vi "configure operation.vi"(7 "tag bus configurable plugin module configuration":refnum<class "io configuration.lvclass">, 8 "error in":errorcluster, 10 "line item in":T3, 11 "engine configuration":refnum<class "engine configuration.lvclass">) -> (0 "error out":errorcluster, 1 "success":bool, 2 "line item out":T3, 5 "changed":bool)   [LabVIEW 2017, in "io editor node.lvclass"]
uses:
  io editor node.lvclass
  table line.ctl
  <vilib>/NI/Tag Bus Module Framework/channel/TBM channel.lvclass
  C:/Program Files (x86)/National Instruments/LabVIEW 2017/vi.lib/NI/Tag Bus/tag/tag descriptor.lvclass
  <vilib>/NI/Module Execution Interface/Engine Configuration/engine configuration.lvclass
  permissions.ctl
  configuration/io configuration.lvclass
  C:/Program Files (x86)/National Instruments/LabVIEW 2017/vi.lib/NI/Configuration Framework/serializable configuration/NISE_CEF_serializable configuration.lvclass
  source/fifo channel/fifo channel settings.ctl
  source/fifo channel/fifo channel.lvclass
  C:/Program Files (x86)/National Instruments/LabVIEW 2017/vi.lib/NI/Tag Bus Module Framework/channel/TBM channel.lvclass
  source/fifo channel/fifo channel.lvclass/fifo channel.ctl
  <vilib>/NI/Tag Bus Module Framework/channel/TBM channel.lvclass/TBM channel.ctl
  <vilib>/NI/Tag Bus/tag/tag descriptor.lvclass/tag descriptor.ctl
  <vilib>/NI/Configuration Framework/serializable configuration/NISE_CEF_serializable configuration.lvclass/NISE_CEF_serializable configuration.ctl
  source/fifo channel/Read fifo config.vi
  <vilib>/NI/Tag Bus Module Framework/channel/Read channel classification.vi
  <vilib>/NI/Tag Bus/tag/read data type.vi
  <vilib>/NI/Configuration Framework/serializable configuration/Read UID.vi
  <vilib>/NI/Tag Bus/tag/write tag name.vi
  source/fifo channel/Write fifo config.vi
  <vilib>/NI/Tag Bus/tag/write data type.vi
  <vilib>/NI/Tag Bus Module Framework/channel/Write channel classification.vi
  <vilib>/Utility/LVClass/Get LV Class Name.vi
  <vilib>/NI/Configuration Framework/error generator/NISE_error generator.vi
  <vilib>/NI/Tag Bus/tag/tag descriptor.lvclass
panel:
  in  "fifo config":T1
  out "errors":string
  in  "Access Type":T2
  in  "Tag":i32(listbox)
  in  "Data Type":i32(listbox)
  in  "Terminal Label":string
  in  "cancel":bool
  in  "ok":bool
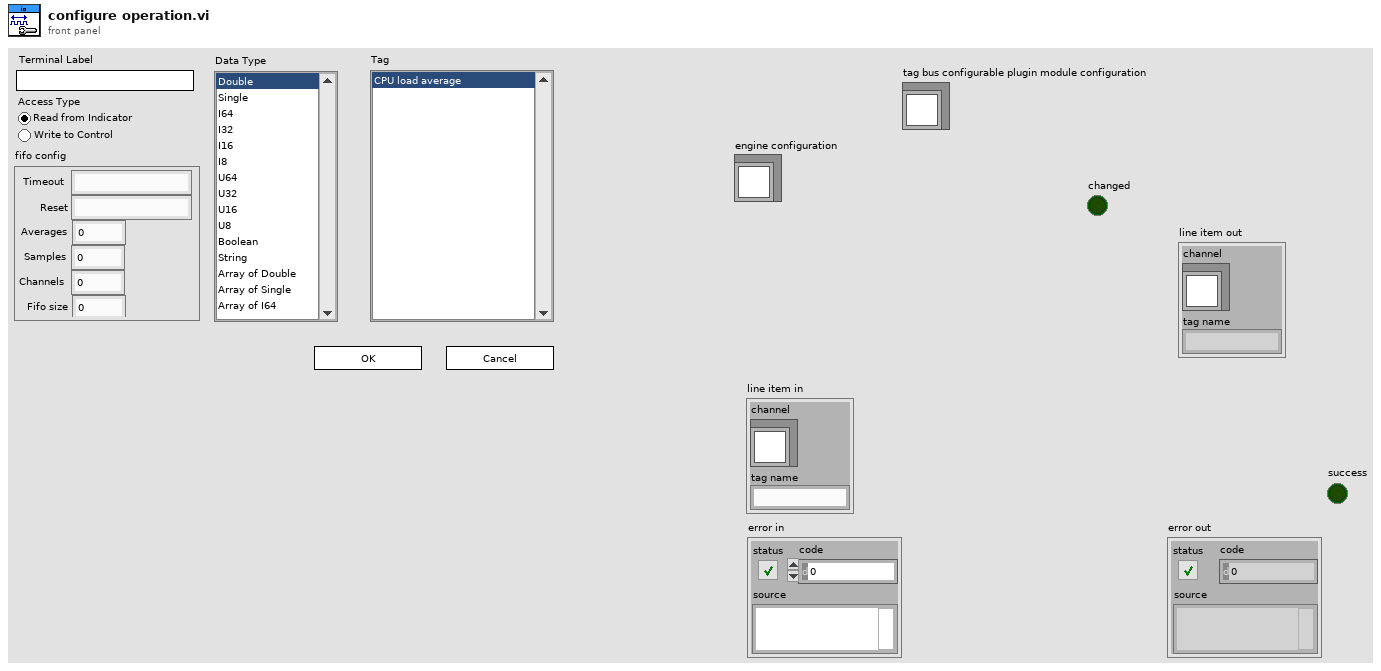
[diagram p1: front panel]
types:
  T1 = typedef "fifo channel.lvclass/fifo channel settings.ctl" = cluster{"Timeout":string, "Reset":string, "Averages":i32, "Samples":u32, "Channels":i32, "Fifo size":u32}
  T2 = typedef "io editor node.lvclass/permissions.ctl" = enum32{"Read from Indicator", "Write to Control"}
  T3 = typedef "io editor node.lvclass/table line.ctl" = cluster{"channel":refnum<class "TBM channel.lvclass">, "tag name":string}
  T4 = enum32{"Invalid", "Standard", "Closed", "Hidden", "Minimized", "Maximized"}
  T5 = enum32{"Invalid", "Default", "Floating", "Floating/Auto-Hide", "Modal"}
  T6 = enum8{"Enabled", "Disabled", "Disabled and Grayed Out"}
  T7 = enum32{"invalid app kind", "Development System", "Run Time System", "Student Edition", "Embedded LabVIEW", "Evaluation", "Custom"}
  T8 = typedef "tag bus.lvlib/tag descriptor.lvclass/Data Type.ctl" = enum16{"Double", "Single", "I64", "I32", "I16", "I8", "U64", "U32", "U16", "U8", "Boolean", "String", "Array of Double", "Array of Single", "Array of I64", "Array of I32", "Array of I16", "Array of I8", "Array of U64", "Array of U32", "Array of U16", "Array of U8", "Array of Boolean", "Array of String"}
  T9 = typedef "TBM channel.lvclass/channel classification.ctl" = enum16{"input data", "output data", "processing parameter", "processing result"}
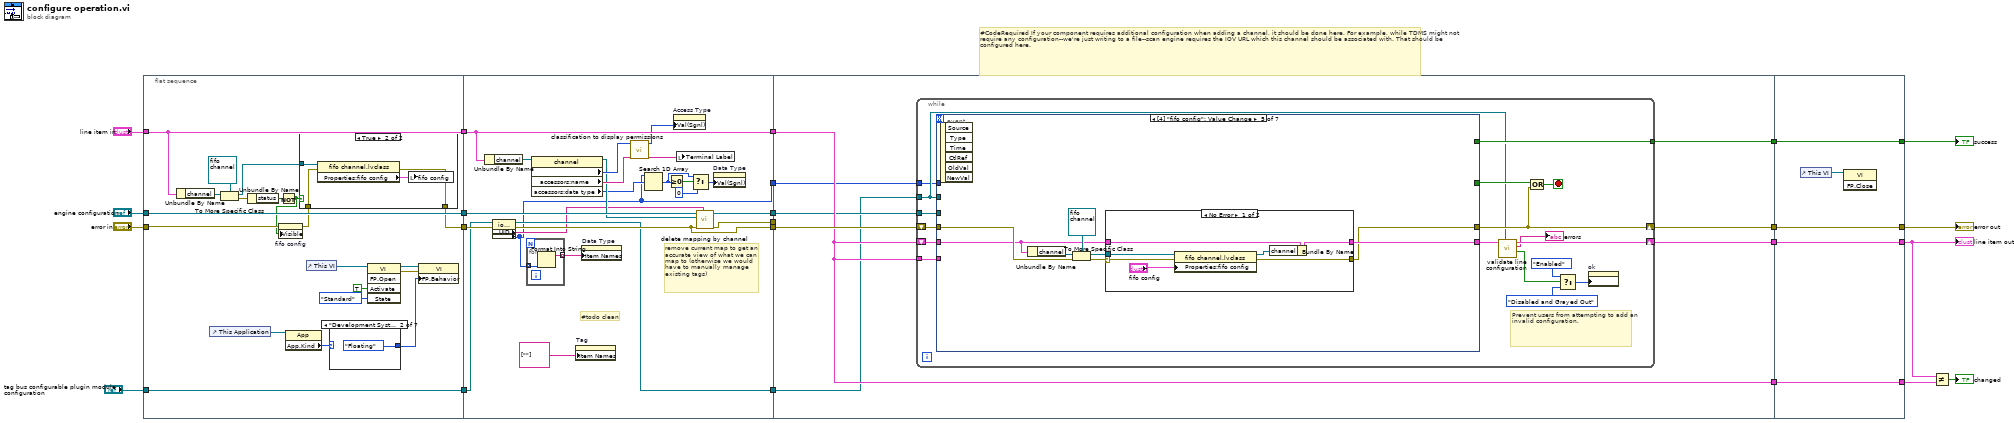
[diagram p0: block diagram]
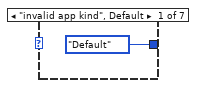
[diagram p3: hidden frame]
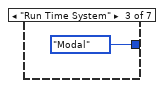
[diagram p4: hidden frame]
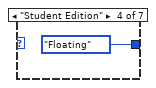
[diagram p5: hidden frame]
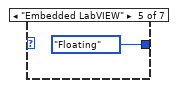
[diagram p6: hidden frame]
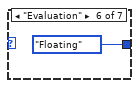
[diagram p7: hidden frame]
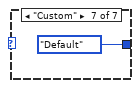
[diagram p8: hidden frame]
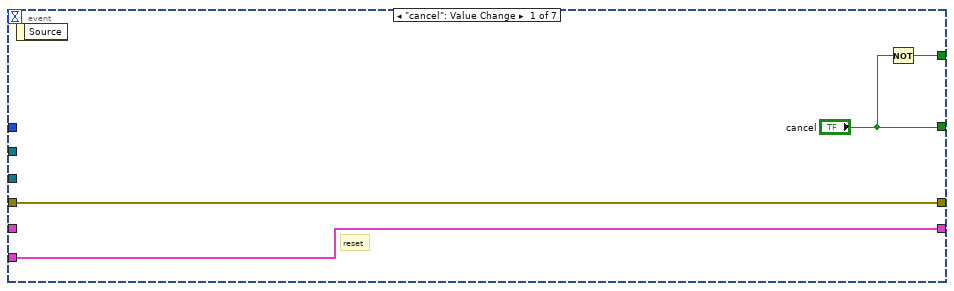
[diagram p9: hidden frame]
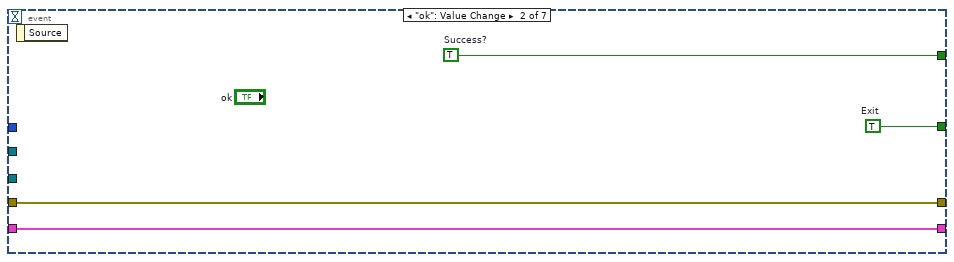
[diagram p10: hidden frame]
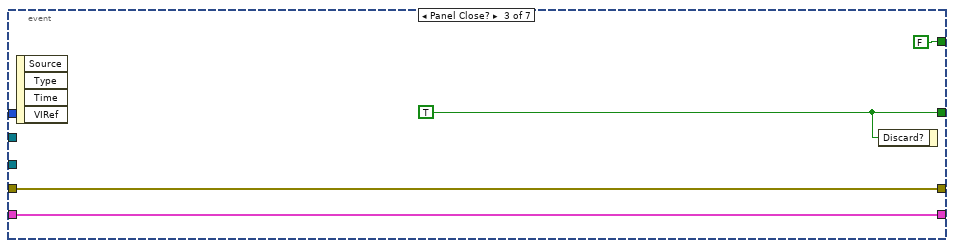
[diagram p11: hidden frame]
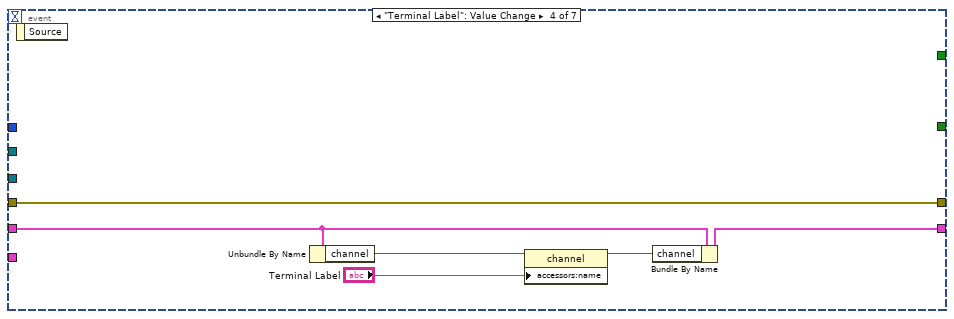
[diagram p12: hidden frame]
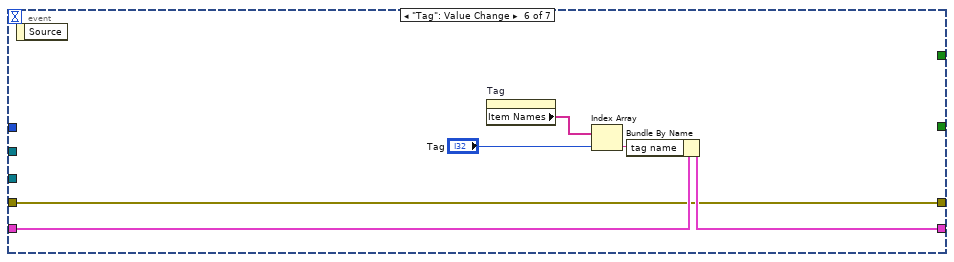
[diagram p14: hidden frame]
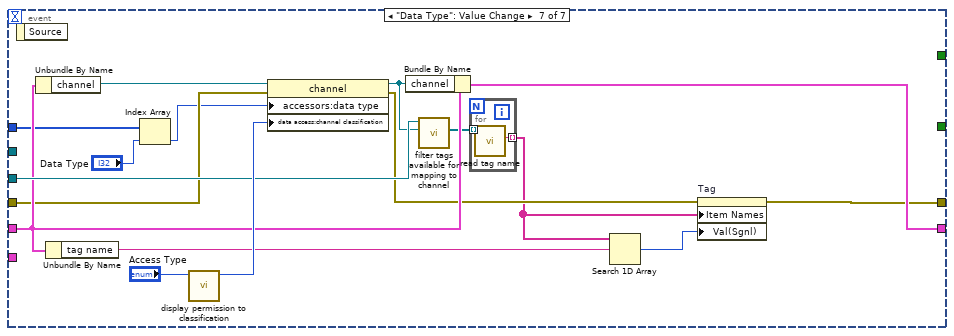
[diagram p15: hidden frame]
diagram:
  # "#CodeRequired If your component requires additional configuration when adding a channel, it should be done here. For example, while TDMS might not require any configuration--we're just writing to a file--scan engine requires the IOV URL which this channel should be associated with. That should be configured here."
  n1 = flat-sequence {
    tunnel: "line item in" -> [w33]
    tunnel: "error in" -> [w26]
    tunnel: [w28] -> w12
    tunnel: [w33] -> w11
    tunnel: [w35] -> w8
    tunnel: "engine configuration" -> [w35]
    tunnel: [w34] -> w5
    tunnel: "tag bus configurable plugin module configuration" -> [w34]
    tunnel: w12 -> [w69]
    tunnel: w11 -> [w74]
    tunnel: [w74] -> w10
    tunnel: [w72] -> w9
    tunnel: w8 -> [w73]
    tunnel: [w66] -> w6
    tunnel: w5 -> [w67]
    tunnel: [w68] -> w4
    tunnel: [w70] -> w3
    tunnel: [w56] -> w2
    tunnel: [w86] -> w16
    tunnel: [w85] -> w15
    tunnel: [w84] -> w14
    tunnel: [w83] -> w13
    tunnel: w10 -> [w83]
    tunnel: w9 -> [w82]
    tunnel: w6 -> [w81]
    tunnel: w4 -> [w87]
    tunnel: w3 -> [_]
    tunnel: w2 -> [w80]
    tunnel: [w166] -> w17
    tunnel: [w167] -> w20
    tunnel: [w168] -> w21
    tunnel: [w169] -> w22
    tunnel: w16 -> [w169]
    tunnel: w15 -> [w168]
    tunnel: w14 -> [w167]
    tunnel: w13 -> [w166]
    frame #0 {
      n2 = Unbundle By Name(w33) -> ("channel"=w32:refnum<class "TBM channel.lvclass">)
      n3 = control-ref of="This Application"() -> (w38:refnum<vi>)
      n4 = To More Specific Class(target class=refnum<class "fifo channel.lvclass"> refnum ("fifo channel.lvclass"), reference=w32) -> (specific class reference=w27:refnum<class "fifo channel.lvclass">, error out=w30:errorcluster)  [unwired: 1 in]
      n5 = Unbundle By Name(w30) -> ("status"=w29:bool)
      n6 = Not(x=w29) -> (.not. x?=w24:bool)
      n7 = property on="fifo config" class="Clust (strict)"(error in=w26, "Visible"=w24) -> (error out=w25:errorcluster)  [unwired: 1 in, 1 out]
      n8 = property class="App"(reference=w38) -> ("App.Kind"=w37:T7)  [unwired: 1 in, 2 out]
      n9 = case shown="True" w24 {
        tunnel: w25 -> [w44 w47]
        tunnel: [w44 w45] -> w28
        tunnel: w27 -> [_ w48]
        frame False {
        }
        frame True {
          n10 = property class="fifo channel.lvclass"(reference=w48, error in=w47) -> (error out=w45:errorcluster, "Properties:fifo config"=w46:T1)  [unwired: 1 out]
          n11 = local write "fifo config"(w46) -> ()
        }
      }
      n12 = control-ref of="This VI"() -> (w39:refnum<vi>)
      n13 = case shown="\"Development System\"" w37 {
        tunnel: [T5."Default" ("Front Panel Window:Behavior") T5."Floating" ("Front Panel Window:Behavior") T5."Modal" ("Front Panel Window:Behavior") T5."Floating" ("Front Panel Window:Behavior") T5."Floating" ("Front Panel Window:Behavior") T5."Floating" ("Front Panel Window:Behavior") T5."Default" ("Front Panel Window:Behavior")] -> w36
        frame "invalid app kind", Default {
        }
        frame "Development System" {
        }
        frame "Run Time System" {
        }
        frame "Student Edition" {
        }
        frame "Embedded LabVIEW" {
        }
        frame "Evaluation" {
        }
        frame "Custom" {
        }
      }
      n14 = invoke class="VI" method="FP.Open"(reference=w39, "Activate"=TRUE ("Activate?"), "State"=T4."Standard") -> (reference out=w42:refnum<vi>, error out=w43:errorcluster)  [unwired: 2 in, 3 out]
      n15 = property class="VI"(reference=w42, error in=w43, "FP.Behavior"=w36) -> ()  [unwired: 2 out]
    }
    frame #1 {
      # "#todo clean"
      # "remove current map to get an accurate view of what we can map to (otherwise we would have to manually manage existing tags)"
      n16 = Unbundle By Name(w74) -> ("channel"=w75:refnum<class "TBM channel.lvclass">)
      n17 = property class="io configuration"(reference=w67, error in=w69) -> (reference out=w66:refnum<class "io configuration.lvclass">, error out=w68:errorcluster, "Properties:UID"=w65:string, "Properties:supported types"=w56:T8[])
      n18 = for {
        tunnel: w56 -> [w79] mode=indexing
        tunnel: [w78] -> w64 mode=indexing
        n19 = Format Into String(w79) -> (resulting string=w78:string)  [unwired: 3 in, 1 out]
      }
      n20 = property class="channel"(reference=w75) -> (reference out=w71:refnum<class "TBM channel.lvclass">, "data access:channel classification"=w77:T9, "accessors:name"=w76:string, "accessors:data type"=w57:T8)  [unwired: 1 in, 1 out]
      n21 = property on="Tag" class="LstBox (strict)"("Item Names"=string[] [""]) -> ()  [unwired: 2 in, 2 out]
      n22 = property on="Data Type" class="LstBox (strict)"("Item Names"=w64) -> ()  [unwired: 2 in, 2 out]
      n23 = call "classification to display permissions.vi"("channel classification"=w77) -> ("permissions"=w58:T2)  [unwired: 10 in]
      n24 = Search 1D Array(1D array=w56, element=w57) -> (index of element=w62:i32)  [unwired: 1 in]
      n25 = Greater Or Equal To 0?(x=w62) -> (x >= 0?=w63:bool)
      n26 = property on="Access Type" class="RadioBtnsControl (strict)"("Val(Sgnl)"=w58) -> ()  [unwired: 2 in, 2 out]
      n27 = local write "Terminal Label"(w76) -> ()
      n28 = Select(t=w62, s=w63, f=0) -> (s? t:f=w60:i32)
      n29 = call <vilib>:"delete mapping by channel.vi"("owner ID"=w65, "error in"=w68, "channel"=w71, "engine configuration in"=w73) -> ("error out"=w70:errorcluster, "engine configuration out"=w72:refnum<class "engine configuration.lvclass">)  [unwired: 6 in]
      n30 = property on="Data Type" class="LstBox (strict)"("Val(Sgnl)"=w60) -> ()  [unwired: 2 in, 2 out]
    }
    frame #2 {
      n31 = while {
        shift-right: [w95] -> w85
        shift-left: w87 -> [w103]
        tunnel: [w102] -> w86
        shift-right: [w96] -> w84
        shift-left: w83 -> [w99]
        tunnel: w83 -> [w98]
        tunnel: w82 -> [w104]
        tunnel: w81 -> [w90]
        tunnel: w80 -> [w89]
        stop <- w100 stop-if-true
        # "Prevent users from attempting to add an invalid configuration."
        n32 = event shown="[4] \"fifo config\": Value Change" {
          selector: _ -> [_ _ _ _ _ _ _]
          dyn-events: _ -> [_ _ _ _ _ _ _]
          timeout: _ -> [_ _ _ _ _ _ _]
          tunnel: w104 -> [_ _ _ _ _ _ w160]
          tunnel: w103 -> [w108 w112 w116 w122 w127 w142 w153]
          tunnel: [w108 w112 w116 w122 w123 w142 w148] -> w95
          tunnel: [w107 w109 FALSE _ _ _ _] -> w102
          tunnel: ["cancel" w110 w114 _ _ _ _] -> w101
          tunnel: w99 -> [_ w111 w113 w120 w125 w145 w158]
          tunnel: [w105 w111 w113 w121 w124 w144 w157] -> w97
          tunnel: w98 -> [w105 _ _ _ _ _ _]
          tunnel: w90 -> [_ _ _ _ _ _ _]
          tunnel: w89 -> [_ _ _ _ _ _ w152]
          event "cancel": Value Change {
            # "reset"
            n33 = event-data() -> ()  [unwired: 1 in, 1 out]
            n34 = Not(x="cancel") -> (.not. x?=w107:bool)
          }
          event "ok": Value Change {
            w109 = TRUE  # Success?
            w110 = TRUE  # Exit
            n35 = event-data() -> ()  [unwired: 1 in, 1 out]
          }
          event Panel Close? {
            w114 = TRUE ("cancel")
            n36 = event-data() -> ()  [unwired: 1 in, 4 out]
            n37 = event-data("Discard?"=w114) -> ()  [unwired: 1 in, 1 out]
          }
          event "Terminal Label": Value Change {
            n38 = event-data() -> ()  [unwired: 1 in, 1 out]
            n39 = Unbundle By Name(w120) -> ("channel"=w119:refnum<class "TBM channel.lvclass">)
            n40 = property class="channel"(reference=w119, "accessors:name"="Terminal Label") -> (reference out=w118:refnum<class "TBM channel.lvclass">)  [unwired: 1 in, 1 out]
            n41 = Bundle By Name(cluster=w120, "channel"=w118) -> (w121:T3)
          }
          event Value Change {
            n42 = event-data() -> ()  [unwired: 1 in, 6 out]
            n43 = Unbundle By Name(w125) -> ("channel"=w130:refnum<class "TBM channel.lvclass">)
            n44 = To More Specific Class(target class=refnum<class "fifo channel.lvclass"> refnum ("fifo channel.lvclass"), reference=w130, error in=w127) -> (specific class reference=w126:refnum<class "fifo channel.lvclass">, error out=w128:errorcluster)
            n45 = case shown="No Error" w128 {
              selector: w128 -> [w133 w138]
              tunnel: w126 -> [w137 _]
              tunnel: w125 -> [w136 w139]
              tunnel: [w135 w139] -> w124
              tunnel: [w131 w138] -> w123
              frame No Error {
                n46 = property class="fifo channel.lvclass"(reference=w137, error in=w133, "Properties:fifo config"="fifo config") -> (reference out=w134:refnum<class "fifo channel.lvclass">, error out=w131:errorcluster)
                n47 = Bundle By Name(cluster=w136, "channel"=w134) -> (w135:T3)
              }
              frame Error {
              }
            }
          }
          event "Tag": Value Change {
            n48 = event-data() -> ()  [unwired: 1 in, 1 out]
            n49 = property on="Tag" class="LstBox (strict)"() -> ("Item Names"=w140:string[])  [unwired: 2 in, 2 out]
            n50 = Index Array(array=w140, index="Tag") -> (element=w143:string)
            n51 = Bundle By Name(cluster=w145, "tag name"=w143) -> (w144:T3)
          }
          event "Data Type": Value Change {
            n52 = event-data() -> ()  [unwired: 1 in, 1 out]
            n53 = Unbundle By Name(w158) -> ("channel"=w162:refnum<class "TBM channel.lvclass">)
            n54 = Unbundle By Name(w158) -> ("tag name"=w155:string)
            n55 = Index Array(array=w152, index="Data Type") -> (element=w150:T8)
            n56 = call "display permission to classification.vi"("display permissions"="Access Type") -> ("channel classification"=w161:T9)  [unwired: 10 in]
            n57 = property class="channel"(reference=w162, error in=w153, "accessors:data type"=w150, "data access:channel classification"=w161) -> (reference out=w159:refnum<class "TBM channel.lvclass">, error out=w149:errorcluster)
            n58 = Bundle By Name(cluster=w158, "channel"=w159) -> (w157:T3)
            n59 = call-dynamic "filter tags available for mapping to channel.vi"("channel to map to"=w159, "engine configuration in"=w160) -> ("filtered tags"=w156:refnum<class "tag descriptor.lvclass">[])  [unwired: 8 in, 1 out]
            n60 = for {
              tunnel: w156 -> [w164] mode=indexing
              tunnel: [w163] -> w147 mode=indexing
              n61 = call <vilib>:"read tag name.vi"("system tag in"=w164) -> ("name"=w163:string)  [unwired: 8 in, 2 out]
            }
            n62 = Search 1D Array(1D array=w147, element=w155) -> (index of element=w146:i32)  [unwired: 1 in]
            n63 = property on="Tag" class="LstBox (strict)"(error in=w149, "Item Names"=w147, "Val(Sgnl)"=w146) -> (error out=w148:errorcluster)  [unwired: 1 in, 1 out]
          }
        }
        n64 = call "validate line configuration.vi"("io configuration"=w90, "line in"=w97) -> ("valid?"=w94:bool, "errors"=→"errors":string, "line out"=w96:T3)  [unwired: 7 in]
        n65 = Compound Arithmetic op=OR(w101, w95) -> (w100:bool)
        n66 = Select(t=T6."Enabled" ("Disabled"), s=w94, f=T6."Disabled and Grayed Out") -> (s? t:f=w91:T6)
        n67 = property on="ok" class="Bool"("DisabledEnum"=w91) -> ()  [unwired: 2 in, 2 out]
      }
    }
    frame #3 {
      n68 = control-ref of="This VI"() -> (w165:refnum<vi>)
      n69 = invoke class="VI" method="FP.Close"(reference=w165) -> ()  [unwired: 2 in, 3 out]
    }
  }
  n70 = Not Equal?(x=w20, y=w17) -> (x != y?=→"changed":bool)
  "error out" <- w21
  "success" <- w22
  "line item out" <- w20
